vi "Send_JSN_Message_1 (SubVI).vi"(6 "id":i32, 9 "data":cluster{"name":string}, 11 "type":string="start") -> (2 "JSON message":string)   [LabVIEW 2015]
uses:
  Ctrl/R_W.ctl
  JSON_conv/Conv_JSON_2 (SubVI).vi
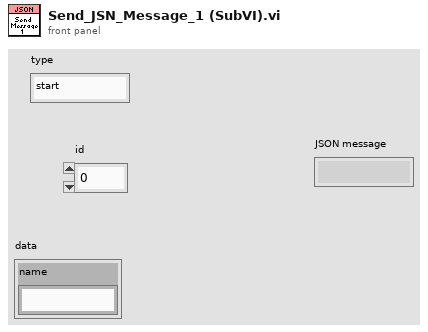
[diagram p1: front panel]
types:
  T1 = cluster{"type":string, "phase":string, "id":u8, "status":i32, "status_msg":string, "device":string}
  T2 = typedef "R_W.ctl" = enum16{"Write", "Read", "RAZ"}
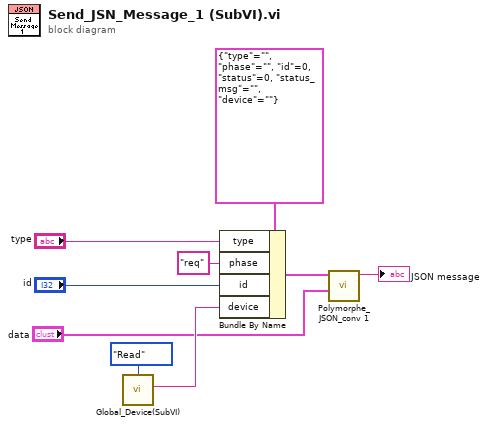
[diagram p0: block diagram]
diagram:
  n1 = call "Global_Device(SubVI).vi"("R/W"=R_W."Read") -> ("Device out"=w9:string)  [unwired: 10 in]
  n2 = Bundle By Name(cluster=T1 {"type"="", "phase"="", "id"=0, "status"=0, "status_msg"="", "device"=""}, "type"="type", "phase"="req", "id"="id", "device"=w9) -> (w4:T1)
  n3 = call-poly "Polymorphe_JSON_conv 1.vi"("data"="data", "Cluster"=w4) -> ("String"=→"JSON message":string)  [unwired: 9 in]
